vi "PH_Beckhoff_PP_PU.declare digital PSU InputTags.vi"(3 "PUs":T1) -> (0 "inverted":bool[](array[boolean]), 1 "Tagnames":string[](array[string]))   [LabVIEW 2014, in "PH_Beckhoff_PP_PU.lvlib"]
uses:
  PH_Beckhoff_PP_PU.lvlib
  PH_Beckhoff_PP_PU.PU Rack Type.ctl
  PH_PP_Common/PH_PP_Common.PSU Tags.ctl
  PH_PP_Common/PH_PP_Common.lvlib
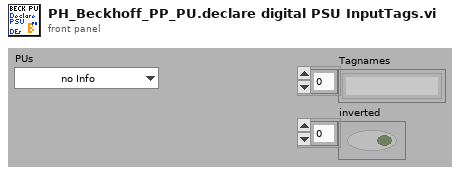
[diagram p1: front panel]
types:
  T1 = typedef "PH_Beckhoff_PP_PU.lvlib/PH_Beckhoff_PP_PU.PU Rack Type.ctl" = enum16{"no Info", "PA 19mm", "PA 45mm", "MA PU 1 and 2", "MA PU 3 and 4", "MA PU 5 and 6", "MA FR and PILC"}
  T2 = typedef "PH_PP_Common.lvlib/PH_PP_Common.PSU Tags.ctl" = enum16{"voltage-indicator", "peak-detect", "current", "voltage", "inihibit-indicator", "end-of-charge", "HV-on-indicator", "overtemperature", "interlock-indicator", "load-fault", "sum-fault", "HV-off-indicator", "DC-ok", "inhibit", "HV-on", "interlock", "reset", "Status", "Limits"}
  T3 = typedef "PH_PP_Common.lvlib/PH_PP_Common.PUs.ctl" = enum16{"no Info", "PA-19mm-1", "PA-19mm-2", "PA-45mm-PILC", "PA-45mm-MAIN", "MA-PU-1", "MA-PU-2", "MA-PU-3", "MA-PU-4", "MA-PU-5", "MA-PU-6", "MA-FR", "MA-PILC", "PA-45mm-DP"}
  T4 = typedef "PH_PP_Common.lvlib/PH_PP_Common.PSU Type.ctl" = enum16{"none", "Maxwell Standard", "DEL", "Maxwell ALE", "Continuum 601k"}
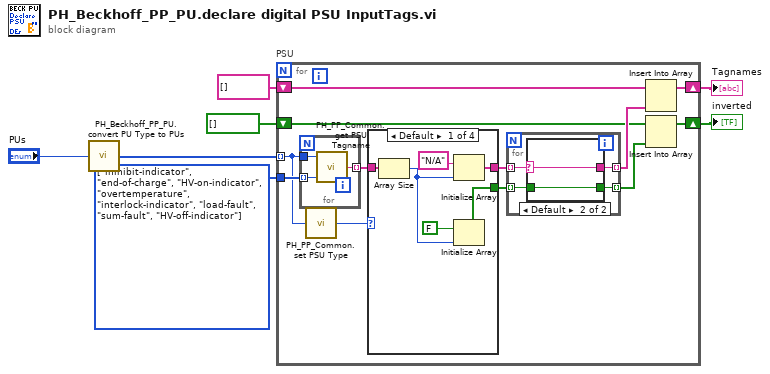
[diagram p0: block diagram]
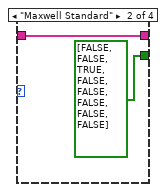
[diagram p2: hidden frame]
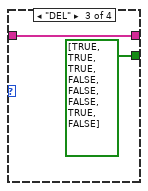
[diagram p3: hidden frame]
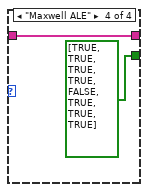
[diagram p4: hidden frame]
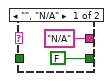
[diagram p5: hidden frame]
diagram:
  w1 = T2[] [enum."inihibit-indicator", enum."end-of-charge", enum."HV-on-indicator", enum."overtemperature", enum."interlock-indicator", enum."load-fault", enum."sum-fault", enum."HV-off-indicator"] items=["voltage-indicator", "peak-detect", "current", "voltage", "inihibit-indicator", "end-of-charge", "HV-on-indicator", "overtemperature", "interlock-indicator", "load-fault", "sum-fault", "HV-off-indicator", "DC-ok", "inhibit", "HV-on", "interlock", "reset", "Status", "Limits"]
  n1 = call "PH_Beckhoff_PP_PU.convert PU Type to PUs.vi"("PU Type"="PUs") -> ("PUs"=w3:T3[])
  n2 = for "PSU" {
    shift-right: [w18] -> w6
    shift-left: string[] [] -> [w17]
    shift-right: [w16] -> w7
    shift-left: bool[] [] -> [w15]
    tunnel: w3 -> [w8] mode=indexing
    tunnel: w1 -> [w10]
    n3 = for {
      tunnel: w8 -> [w22]
      tunnel: w10 -> [w21] mode=indexing
      tunnel: [w20] -> w11 mode=indexing
      n4 = call "PH_PP_Common.get PSU Tagname.vi"("PSU Tag"=w21, "PU"=w22) -> ("PSU Tagname"=w20:string)  [unwired: 1 in]
    }
    n5 = call "PH_PP_Common.set PSU Type.vi"("PU"=w8) -> ("PSU Type"=w9:T4)
    n6 = case shown="Default" w9 {
      tunnel: [w28 w29 w31 w33] -> w13
      tunnel: [w25 bool[] [FALSE, FALSE, TRUE, FALSE, FALSE, FALSE, FALSE, FALSE] bool[] [TRUE, TRUE, TRUE, FALSE, FALSE, FALSE, TRUE, FALSE] bool[] [TRUE, TRUE, TRUE, TRUE, FALSE, TRUE, TRUE, TRUE]] -> w12
      tunnel: w11 -> [w26 w29 w31 w33]
      frame Default {
        n7 = Array Size(array=w26) -> (size(s)=w24:i32)
        n8 = Initialize Array("N/A", w24) -> (w28:string[])
        n9 = Initialize Array(FALSE ("element"), w24) -> (w25:bool[])
      }
      frame "Maxwell Standard" {
      }
      frame "DEL" {
      }
      frame "Maxwell ALE" {
      }
    }
    n10 = for {
      tunnel: [w38] -> w19 mode=indexing
      tunnel: [w37] -> w14 mode=indexing
      tunnel: w13 -> [w36] mode=indexing
      tunnel: w12 -> [w35] mode=indexing
      n11 = case shown="Default" w36 {
        selector: w36 -> [_ w42]
        tunnel: ["N/A" w42] -> w38
        tunnel: w35 -> [_ w41]
        tunnel: [FALSE ("element") w41] -> w37
        frame "", "N/A" {
        }
        frame Default {
        }
      }
    }
    n12 = Insert Into Array(array=w17, new element=w19) -> (w18:string[])  [unwired: 1 in]
    n13 = Insert Into Array(array=w15, new element=w14) -> (w16:bool[])  [unwired: 1 in]
  }
  "inverted" <- w7
  "Tagnames" <- w6
